vi "XAxisInputs (1).vi"(7 "t_s":dbl, 8 "error in (no error)":errorcluster, 9 "t_s@(N-1)":dbl, 10 "Reset Timer and Encoder Counts":bool, 11 "X_Dist_mm@(N-1)":dbl) -> (0 "error out":errorcluster, 2 "X_Dist_mm@(N)":dbl, 3 "X_FiltSpeed(mm/s)":dbl)   [LabVIEW 2013]
uses:
  <vilib>/myRIO/Instrument Drivers/Onboard IO/Encoder/vis/Smart Open.vi
  <vilib>/myRIO/Instrument Drivers/Onboard IO/Encoder/vis/Read.vi
  <vilib>/myRIO/Instrument Drivers/Onboard IO/Encoder/vis/Open.vi
  <vilib>/myRIO/Common/Instrument Driver Framework/myRIO v1.0/Encoder/vis/myRIO v1.1 Open Encoder.vi
  <vilib>/myRIO/Common/Instrument Driver Framework/myRIO v1.0/Encoder/vis/myRIO v1.0 Close Encoder.vi
  <vilib>/myRIO/Common/Instrument Driver Framework/Utilities/vis/Validate Channels.vi
  <vilib>/myRIO/Common/Instrument Driver Framework/myRIO v1.0/Encoder/vis/myRIO v1.0 Reserve Encoder.vi
  <vilib>/myRIO/Common/Instrument Driver Framework/myRIO v1.0/Encoder/vis/myRIO v1.0 Unreserve Encoder.vi
  <vilib>/myRIO/Common/Instrument Driver Framework/myRIO v1.0/Encoder/vis/myRIO v1.0 Build MUX Configuration Encoder.vi
  <vilib>/myRIO/Common/Instrument Driver Framework/myRIO v1.0/Resource Manager/vis/myRIO v1.0 Reserve Channel List.vi
  <vilib>/myRIO/Common/Instrument Driver Framework/myRIO v1.0/Resource Manager/vis/myRIO v1.0 Unreserve Channel List.vi
  <vilib>/myRIO/Common/Instrument Driver Framework/myRIO v1.0/Resource Manager/vis/myRIO v1.0 Create Configuration List.vi
  <vilib>/myRIO/Common/Instrument Driver Framework/myRIO v1.0/Resource Manager/vis/myRIO v1.0 Reserve Channel.vi
  <vilib>/myRIO/Common/Instrument Driver Framework/myRIO v1.0/Resource Manager/vis/myRIO v1.0 Unreserve Channel.vi
  <vilib>/myRIO/Common/Instrument Driver Framework/myRIO v1.0/Resource Manager/vis/myRIO v1.0 Build Mutex Name.vi
  <vilib>/myRIO/Common/Instrument Driver Framework/myRIO v1.0/Encoder/vis/myRIO v1.0 Configure Encoder.vi
  <vilib>/myRIO/Common/Instrument Driver Framework/myRIO v1.0/myRIO v1.1 Open.vi
  <vilib>/Utility/VariantDataType/GetNumericInfo.vi
  <vilib>/Utility/error.llb/Error Cluster From Error Code.vi
  <vilib>/myRIO/Common/Instrument Driver Framework/Utilities/vis/IO Manager.vi
  <vilib>/myRIO/Common/Instrument Driver Framework/Utilities/vis/Configuration Manager.vi
  <vilib>/myRIO/Common/Instrument Driver Framework/myRIO v1.0/Resource Manager/vis/myRIO v1.0 Configure IO.vi
  <vilib>/myRIO/Common/Instrument Driver Framework/myRIO v1.0/myRIO v1.0 Close.vi
  <vilib>/myRIO/Common/Instrument Driver Framework/myRIO v1.0/Encoder/vis/myRIO v1.0 Shutdown Encoder.vi
  <vilib>/myRIO/Common/Instrument Driver Framework/myRIO v1.0/Encoder/vis/myRIO v1.0 Read Encoder.vi
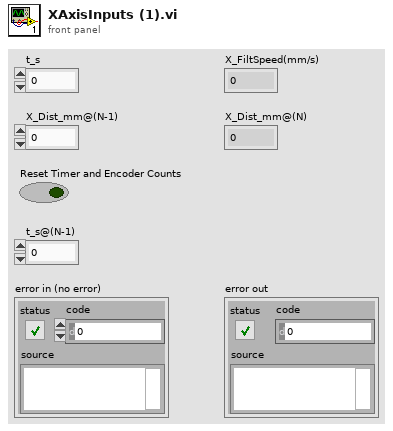
[diagram p1: front panel]
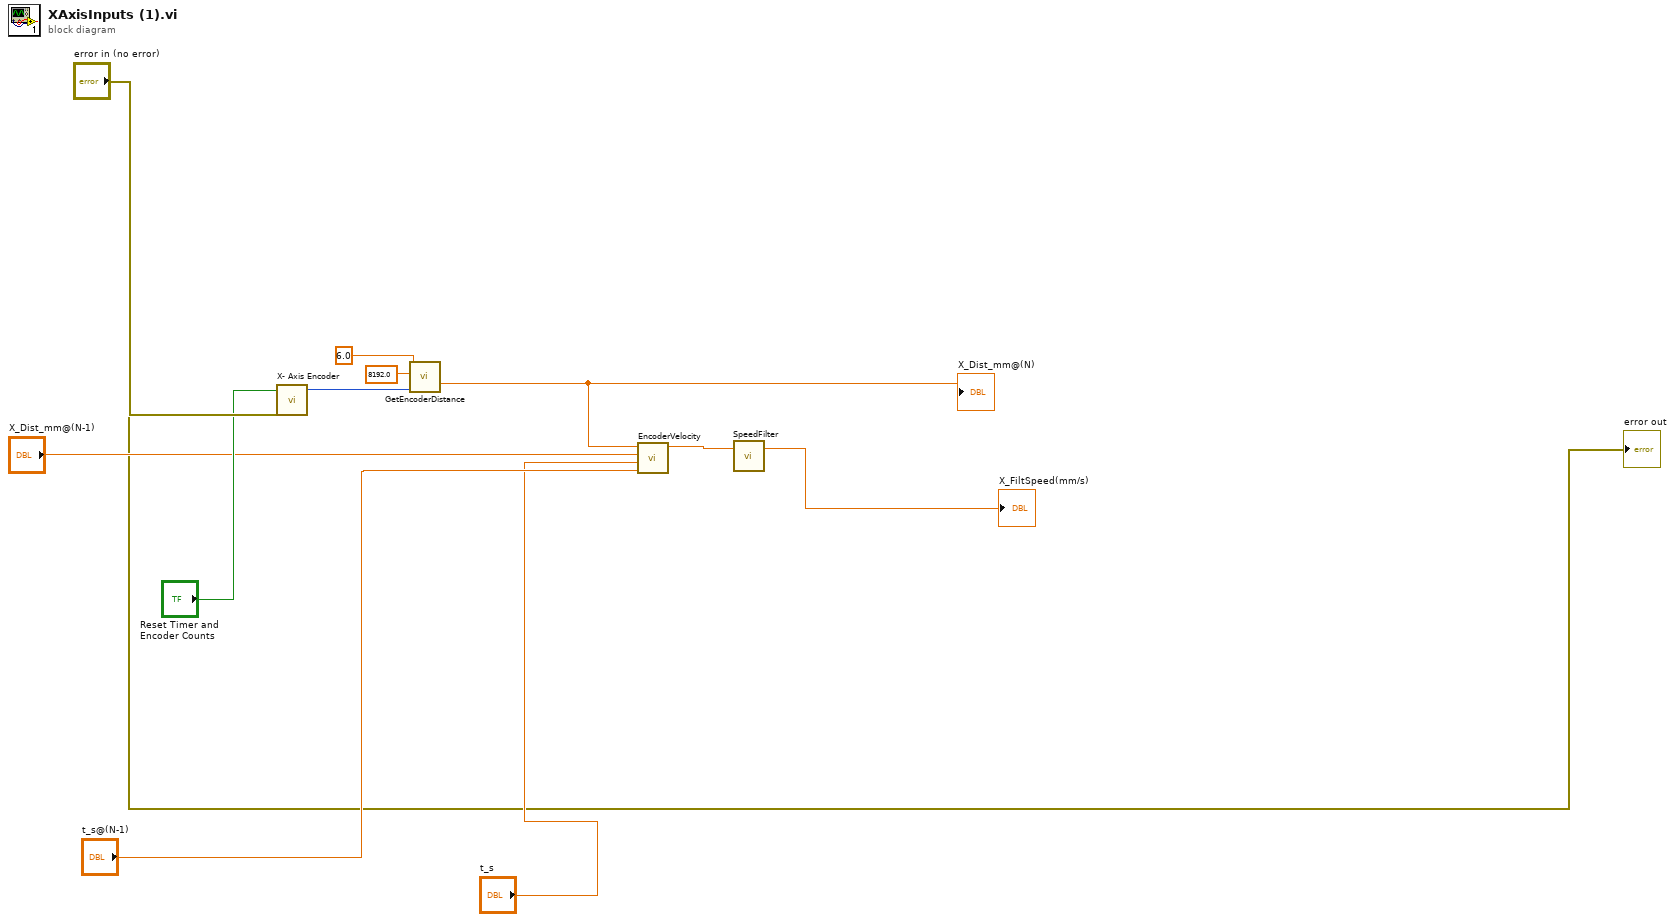
[diagram p0: block diagram]
diagram:
  n1 = call "X- Axis Encoder"("Reset Counter"="Reset Timer and Encoder Counts", "error in (no error)"="error in (no error)") -> ("Counter Value"=w6:i32, "error out"=→"error out":errorcluster)  [unwired: 22 in, 2 out]
  n2 = call "GetEncoderDistance.vi"("Encoder Count"=w6, "Resolution (Counts per rev)"=8192.0, "Lead Screw Lead (mm/rev)"=6.0) -> ("Distance from origin (mm)"=w11:dbl)  [unwired: 8 in]
  "X_Dist_mm@(N)" <- w11
  n3 = call "EncoderVelocity.vi"("Time @(n-1)"="t_s@(N-1)", "Time @n"="t_s", "Encoder Distance (mm) @n-1"="X_Dist_mm@(N-1)", "Encoder Distance (mm) @n"=w11) -> ("Encoder Speed (mm/s)"=w8:dbl)  [unwired: 7 in]
  n4 = call "SpeedFilter.vi"("Raw Signal"=w8) -> ("Filtered Signal"=→"X_FiltSpeed(mm/s)":dbl)  [unwired: 1 in, 1 out]
